vi "Slider Properties.vi"(1 "error in (no error) 2":errorcluster, 2 "Array":refnum<vi>[](array[refnum])) -> (0 "error out":errorcluster)   [LabVIEW 2009]
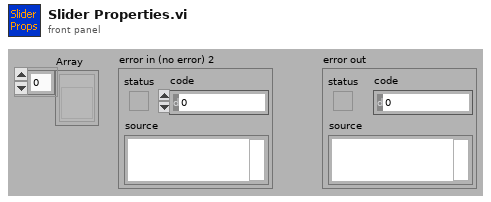
[diagram p1: front panel]
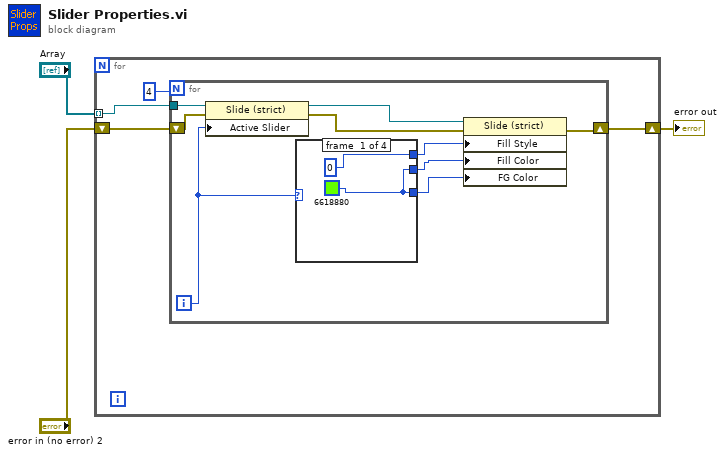
[diagram p0: block diagram]
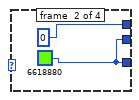
[diagram p2: hidden frame]
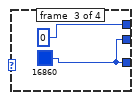
[diagram p3: hidden frame]
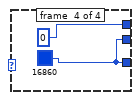
[diagram p4: hidden frame]
diagram:
  n1 = for {
    tunnel: "Array" -> [w7] mode=indexing
    shift-right: [w5] -> w3
    shift-left: "error in (no error) 2" -> [w6]
    n2 = for {
      N: 4 -> [_]
      tunnel: w7 -> [w16]
      shift-right: [w12] -> w5
      shift-left: w6 -> [w10]
      i -> [w8]
      n3 = property class="Slide (strict)"(reference=w16, error in=w10, "Active Slider"=w8) -> (reference out=w11:refnum<vi>, error out=w9:errorcluster)
      n4 = case shown="0, Default" w8 {
        tunnel: [0 ("Fill Style") 0 ("Fill Style") 0 ("Fill Style") 0 ("Fill Style")] -> w15
        tunnel: [w17 w19 w21 w23] -> w14
        tunnel: [w17 w19 w21 w23] -> w13
        frame #0 {
          w17 = u32 6618880 ("Fill Color")
        }
        frame #1 {
          w19 = u32 6618880 ("Fill Color")
        }
        frame #2 {
          w21 = u32 16860 ("Fill Color")
        }
        frame #3 {
          w23 = u32 16860 ("Fill Color")
        }
      }
      n5 = property class="Slide (strict)"(reference=w11, error in=w9, "Fill Style"=w15, "Fill Color"=w14, "FG Color"=w13) -> (error out=w12:errorcluster)  [unwired: 1 out]
    }
  }
  "error out" <- w3
